vi "Pruebas con VISA.vi"() -> ()   [LabVIEW 2019]
uses:
  Controles/Amp_Frec.ctl
  <vilib>/Utility/error.llb/DialogType.ctl
  QMH_Support/Enqueue Message (Single).vi
  Varios/Globales.vi
  <vilib>/Utility/error.llb/Error Cluster From Error Code.vi
  <vilib>/ErrorRing/Error Ring.xnode
  QMH_Support/Message Queue.lvlib
  QMH_Support/User Event - Stop/User Event - Stop.lvlib
  DS360/DS360.lvlib
  K2002/K2002.lvlib
  CNT90/CNT90.lvlib
panel:
  in  "CNT90":refnum<visa-resource-name>
  in  "DS360":refnum<visa-resource-name>
  in  "K2002":refnum<visa-resource-name>
  in  "go_A":bool
  out "CNT90":i32
  out "K2002":i32
  out "DS360":i32
  out "Voltaje a generar":dbl(knob) scale=0.0..10.0
  out "error out":errorcluster
  in  "stop":bool
  in  "generar":bool
  in  "Voltaje a Generar":dbl(slide)=7.0649350649350655 scale=0.0..10.0
  out "voltMon":dbl format="%.2f"
  out "frecMon":dbl format="%.2f"
  # "Ensayo Eléctrico Ponderación A"
  # "Monitoreo"
  # "Frecuencia"
  # "Hz"
  # "Voltaje"
  # "mV"
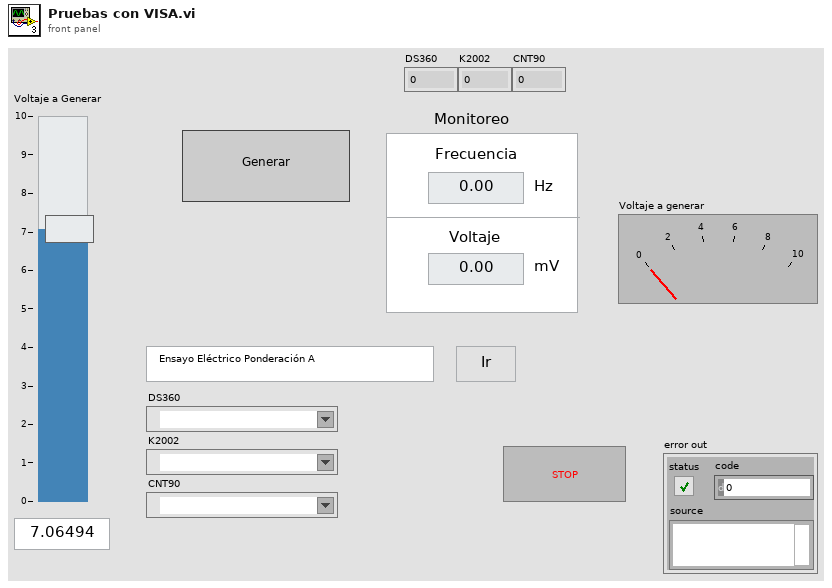
[diagram p1: front panel]
types:
  T1 = typedef "Message Queue.lvlib/All Message Queues.ctl" = cluster{"MHL":refnum<queue>, "DS360":refnum<queue>, "K2002":refnum<queue>, "CNT90":refnum<queue>}
  T2 = typedef "Amp_Frec.ctl" = cluster{"Ampl":dbl, "Frec":dbl}
  T3 = typedef "DialogType.ctl" = u16
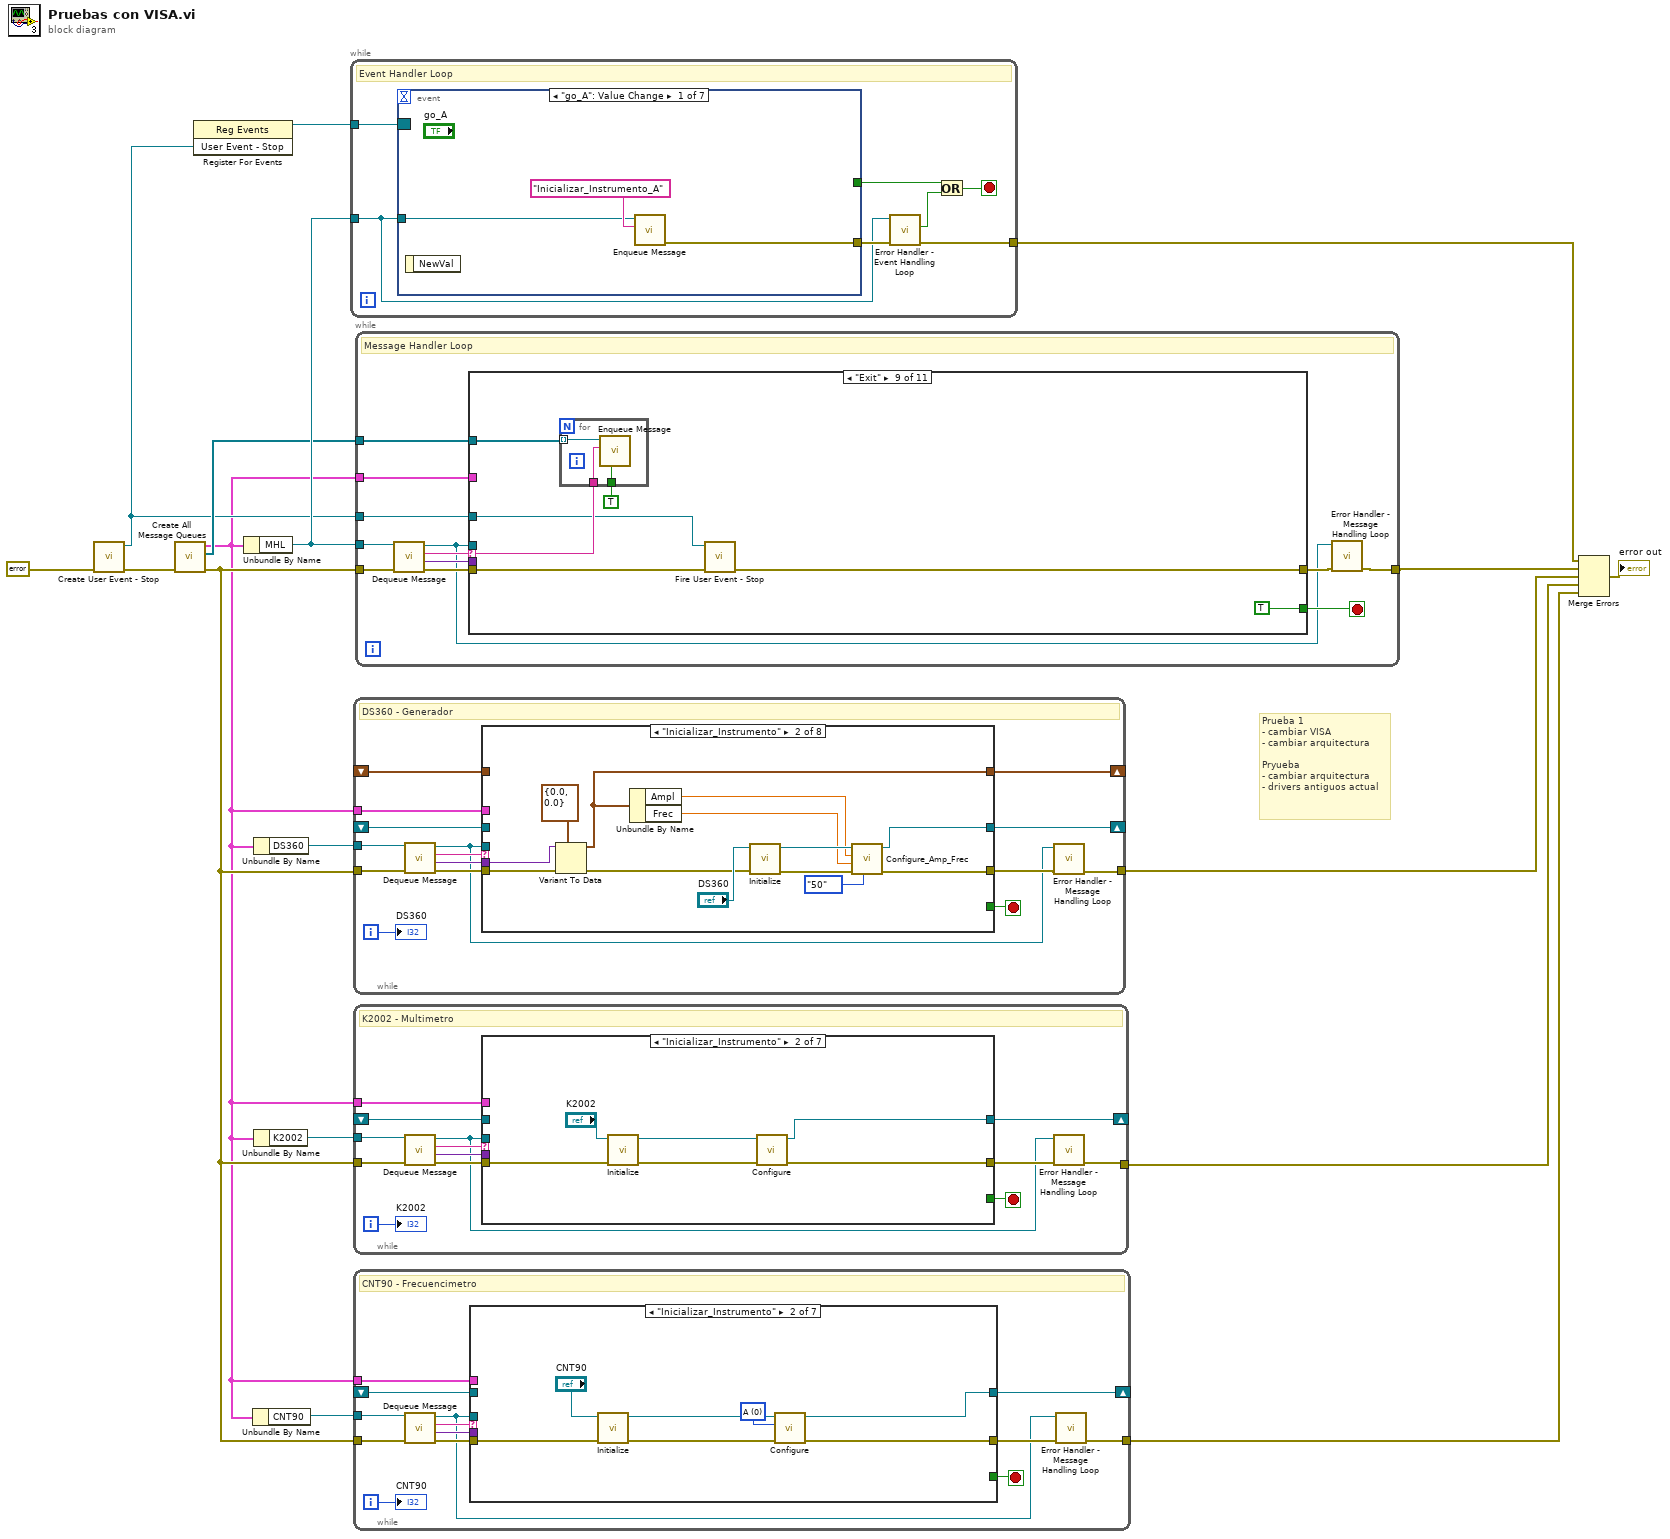
[diagram p0: block diagram]
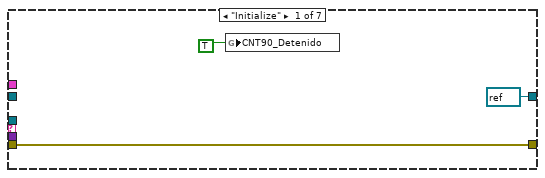
[diagram p2: hidden frame]
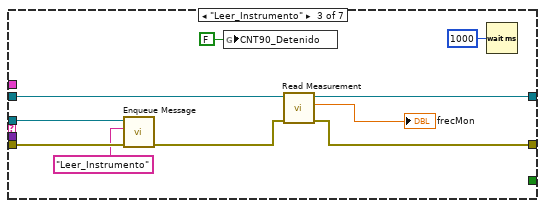
[diagram p3: hidden frame]
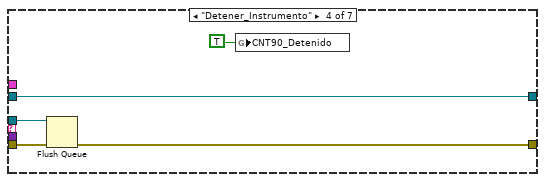
[diagram p4: hidden frame]
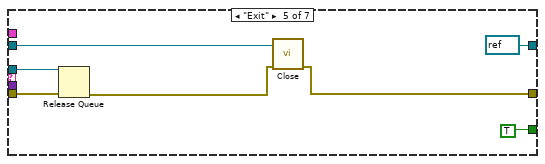
[diagram p5: hidden frame]
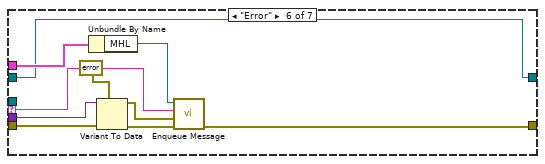
[diagram p6: hidden frame]
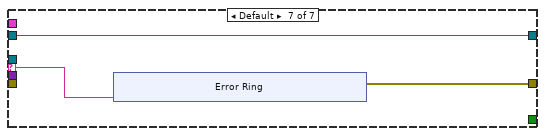
[diagram p7: hidden frame]
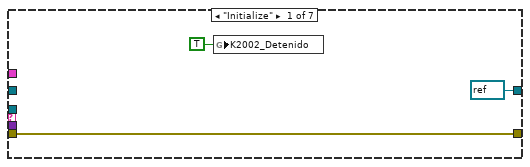
[diagram p8: hidden frame]
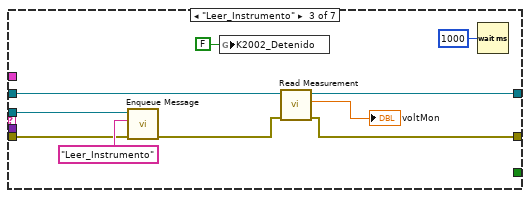
[diagram p9: hidden frame]
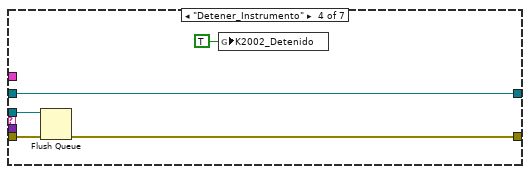
[diagram p10: hidden frame]
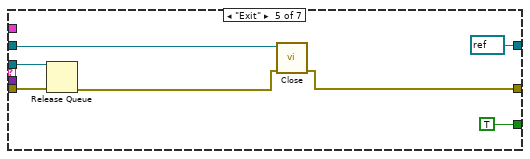
[diagram p11: hidden frame]
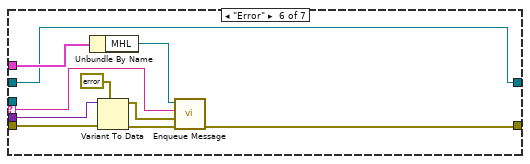
[diagram p12: hidden frame]
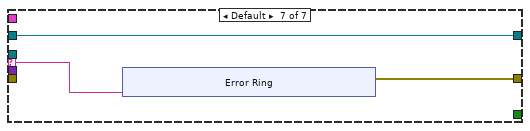
[diagram p13: hidden frame]
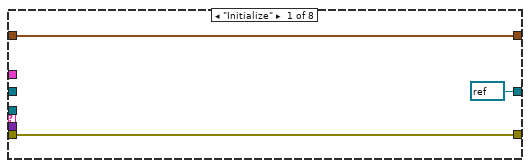
[diagram p14: hidden frame]
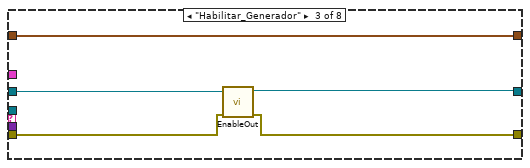
[diagram p15: hidden frame]
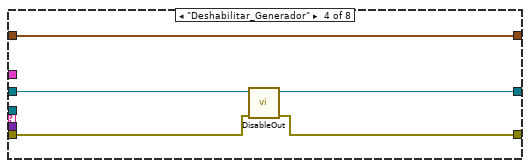
[diagram p16: hidden frame]
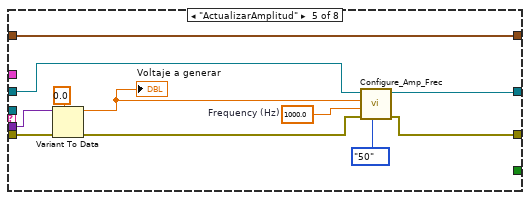
[diagram p17: hidden frame]
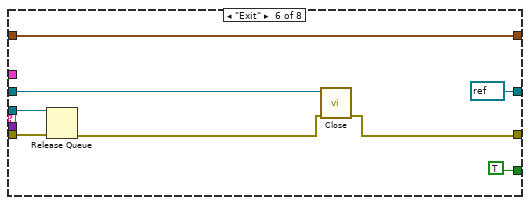
[diagram p18: hidden frame]
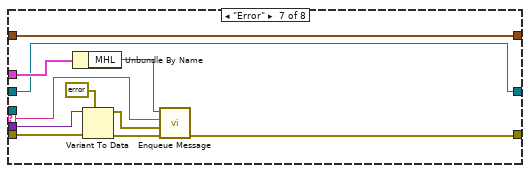
[diagram p19: hidden frame]
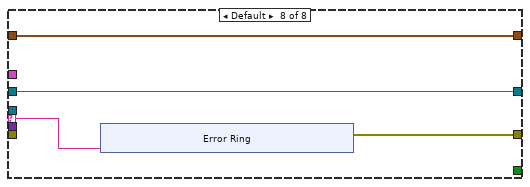
[diagram p20: hidden frame]
diagram:
  # "Prueba 1\n- cambiar VISA\n- cambiar arquitectura\n\nPryueba\n- cambiar arquitectura\n- drivers antiguos actual"
  n1 = call "Create User Event - Stop.vi"("error in (no error)"=errorcluster {"status"=FALSE, "code"=0, "source"=""}) -> ("error out"=w9:errorcluster, "User Event - Stop"=w8:refnum<user-event>)  [unwired: 9 in]
  n2 = call "Create All Message Queues.vi"("error in (no error)"=w9) -> ("error out"=w6:errorcluster, "Queues Array"=w11:refnum<queue>[], "Message Queues out"=w3:T1)  [unwired: 8 in]
  n3 = register-events(w8) -> (reference out=w7:refnum<event-registration>)  [unwired: 2 in, 1 out]
  n4 = Unbundle By Name(w3) -> ("MHL"=w17:refnum<queue>)
  n5 = Unbundle By Name(w3) -> ("CNT90"=w4:refnum<queue>)
  n6 = Unbundle By Name(w3) -> ("DS360"=w16:refnum<queue>)
  n7 = Unbundle By Name(w3) -> ("K2002"=w5:refnum<queue>)
  n8 = while {
    tunnel: w17 -> [w21]
    tunnel: [w22] -> w15
    tunnel: w7 -> [w24]
    stop <- w18 stop-if-true
    # "Event Handler Loop"
    n9 = event shown="[0] \"go_A\": Value Change" {
      selector: w24 -> [_ _ _ _ _ _ _]
      dyn-events: _ -> [_ _ _ _ _ _ _]
      timeout: _ -> [_ _ _ _ _ _ _]
      tunnel: w21 -> [w26 w29 w38 w46 w51 w59 _]
      tunnel: [w25 w28 w39 w45 w52 w57 _] -> w23
      tunnel: [_ _ _ _ _ _ TRUE] -> w20
      event "go_A": Value Change {
        n10 = event-data() -> ()  [unwired: 1 in, 1 out]
        n11 = call-poly "Enqueue Message.vi"("Message"="Inicializar_Instrumento_A" ("message"), "Message Queue"=w26) -> ("error out"=w25:errorcluster)  [unwired: 8 in, 1 out]
      }
      event "generar": Value Change {
        n12 = event-data() -> ("NewVal"=w30:bool)  [unwired: 1 in]
        n13 = Flush Queue(queue=w29) -> (queue out=w31:refnum<queue>, error out=w32:errorcluster)  [unwired: 1 in, 1 out]
        n14 = Select(t="iniciarGEN_A1" ("message"), s=w30, f="detenerGEN" ("message")) -> (s? t:f=w35:string)
        n15 = call-poly "Enqueue Message.vi"("Priority Message? (F)"=TRUE, "error in (no error)"=w32, "Message Data"="A1" ("message"), "Message"=w35, "Message Queue"=w31) -> ("error out"=w28:errorcluster)  [unwired: 5 in, 1 out]
      }
      event "Voltaje a Generar": Mouse Down {
        n16 = event-data() -> ()  [unwired: 1 in, 1 out]
        n17 = Flush Queue(queue=w38) -> (queue out=w40:refnum<queue>, error out=w41:errorcluster)  [unwired: 1 in, 1 out]
        n18 = call-poly "Enqueue Message.vi"("Priority Message? (F)"=TRUE, "error in (no error)"=w41, "Message"="Mouse_Down" ("message"), "Message Queue"=w40) -> ("error out"=w39:errorcluster)  [unwired: 6 in, 1 out]
      }
      event "Voltaje a Generar": Value Change {
        n19 = event-data() -> ("NewVal"=w44:dbl)  [unwired: 1 in]
        n20 = Flush Queue(queue=w46) -> (queue out=w47:refnum<queue>, error out=w48:errorcluster)  [unwired: 1 in, 1 out]
        n21 = call-poly "Enqueue Message.vi"("Priority Message? (F)"=TRUE, "error in (no error)"=w48, "Message Data"=w44, "Message"="EnviarVoltajeGEN" ("message"), "Message Queue"=w47) -> ("error out"=w45:errorcluster)  [unwired: 5 in, 1 out]
      }
      event "Voltaje a Generar": Mouse Up {
        n22 = event-data() -> ()  [unwired: 1 in, 1 out]
        n23 = Flush Queue(queue=w51) -> (queue out=w53:refnum<queue>, error out=w54:errorcluster)  [unwired: 1 in, 1 out]
        n24 = call-poly "Enqueue Message.vi"("Priority Message? (F)"=TRUE, "error in (no error)"=w54, "Message"="Reiniciar_Lectura" ("message"), "Message Queue"=w53) -> ("error out"=w52:errorcluster)  [unwired: 6 in, 1 out]
      }
      event "stop": Value Change {
        n25 = event-data() -> ()  [unwired: 1 in, 1 out]
        n26 = call-poly "Enqueue Message.vi"("Message"="Exit", "Message Queue"=w59) -> ("error out"=w57:errorcluster)  [unwired: 8 in, 1 out]
      }
      event User Event {
        n27 = event-data() -> ()  [unwired: 1 in, 1 out]
      }
    }
    n28 = call "Error Handler - Event Handling Loop.vi"("error in (no error)"=w23, "Message Queue"=w21) -> ("dup error in"=w22:errorcluster, "Error?"=w19:bool)  [unwired: 7 in, 1 out]
    n29 = Or(x=w20, y=w19) -> (x .or. y?=w18:bool)
  }
  n30 = while {
    tunnel: w16 -> [w75]
    tunnel: w6 -> [w74]
    tunnel: [w62] -> w13
    tunnel: w3 -> [w70]
    shift-right: [w67] -> _
    shift-left: _ -> [w66]
    shift-right: [w65] -> _
    shift-left: _ -> [w64]
    i -> [w68]
    stop <- w69 stop-if-true
    # "DS360 - Generador"
    n31 = call "Dequeue Message.vi"("error in (no error)"=w74, "Message Queue"=w75) -> ("error out"=w73:errorcluster, "Message Data"=w71:variant, "Message"=w72:string, "dup Message Queue"=w61:refnum<queue>)  [unwired: 6 in]
    n32 = case shown="\"Inicializar_Instrumento\"" w72 {
      selector: w72 -> [_ _ _ _ _ _ w124 w135]
      tunnel: w73 -> [w77 w91 w95 w98 w111 w120 w127 _]
      tunnel: w71 -> [_ w89 _ _ w110 _ w126 _]
      tunnel: w61 -> [_ _ _ _ _ w119 _ _]
      tunnel: [w77 w84 w94 w97 w107 w113 w123 w134] -> w63
      tunnel: w70 -> [_ _ _ _ _ _ w125 _]
      tunnel: [_ _ _ _ _ TRUE _ _] -> w69
      tunnel: [w78 w88 w96 w101 w109 w117 w122 w133] -> w67
      tunnel: w66 -> [w78 _ w96 w101 w109 w117 w122 w133]
      tunnel: [refnum<visa-resource-name> refnum ("VISA resource name out") w80 w92 w99 w106 refnum<visa-resource-name> refnum ("VISA resource name out") w121 w132] -> w65
      tunnel: w64 -> [_ _ w93 w100 w105 w116 w121 w132]
      frame "Initialize" {
      }
      frame "Inicializar_Instrumento" {
        n33 = Variant To Data(error in=w91, type=T2 {"Ampl"=0.0, "Frec"=0.0}, Variant=w89) -> (data=w88:T2, error out=w86:errorcluster)
        n34 = Unbundle By Name(w88) -> ("Ampl"=w82:dbl, "Frec"=w81:dbl)
        n35 = call "Initialize.vi"("error in (no error)"=w86, "VISA resource name"="DS360") -> ("error out"=w85:errorcluster, "VISA resource name out"=w83:refnum<visa-resource-name>)  [unwired: 8 in]
        n36 = call "Configure_Amp_Frec.vi"("Impedancia"=enum16{"50", "600", "HiZ"}."50", "error in (no error)"=w85, "Frequency (Hz)"=w81, "Amplitude (Vrms)"=w82, "VISA resource name"=w83) -> ("error out"=w84:errorcluster, "VISA resource name out"=w80:refnum<visa-resource-name>)  [unwired: 5 in]
      }
      frame "Habilitar_Generador" {
        n37 = call "EnableOut.vi"("error in (no error)"=w95, "VISA resource name"=w93) -> ("error out"=w94:errorcluster, "VISA resource name out"=w92:refnum<visa-resource-name>)  [unwired: 8 in]
      }
      frame "Deshabilitar_Generador" {
        n38 = call "DisableOut.vi"("error in (no error)"=w98, "VISA resource name"=w100) -> ("error out"=w97:errorcluster, "VISA resource name out"=w99:refnum<visa-resource-name>)  [unwired: 8 in]
      }
      frame "ActualizarAmplitud" {
        w103 = 1000.0  # Frequency (Hz)
        n39 = Variant To Data(error in=w111, type=0.0, Variant=w110) -> (data=w104:dbl, error out=w108:errorcluster)
        "Voltaje a generar" <- w104
        n40 = call "Configure_Amp_Frec.vi"("Impedancia"=enum16{"50", "600", "HiZ"}."50", "error in (no error)"=w108, "Frequency (Hz)"=w103, "Amplitude (Vrms)"=w104, "VISA resource name"=w105) -> ("error out"=w107:errorcluster, "VISA resource name out"=w106:refnum<visa-resource-name>)  [unwired: 5 in]
      }
      frame "Exit" {
        n41 = Release Queue(queue=w119, error in (no error)=w120) -> (error out=w114:errorcluster)  [unwired: 1 in, 2 out]
        n42 = call "Close.vi"("error in (no error)"=w114, "VISA resource name"=w116) -> ("error out"=w113:errorcluster)  [unwired: 9 in]
      }
      frame "Error" {
        n43 = Unbundle By Name(w125) -> ("MHL"=w128:refnum<queue>)
        n44 = Variant To Data(error in=w127, type=errorcluster {"status"=FALSE, "code"=0, "source"=""} ("error constant"), Variant=w126) -> (data=w129:errorcluster, error out=w130:errorcluster)
        n45 = call-poly "Enqueue Message.vi"("error in (no error)"=w130, "Message Data"=w129, "Message"=w124, "Message Queue"=w128) -> ("error out"=w123:errorcluster)  [unwired: 6 in, 1 out]
      }
      frame Default {
        n46 = xnode "Error Ring"("parameter 0"=w135) -> ("error out"=w134:errorcluster)
      }
    }
    n47 = call "Error Handler - Message Handling Loop.vi"("error in (no error)"=w63, "Message Queue"=w61) -> ("dup error in"=w62:errorcluster)  [unwired: 8 in, 1 out]
    "DS360" <- w68
  }
  n48 = while {
    tunnel: w5 -> [w155]
    tunnel: w6 -> [w154]
    tunnel: w3 -> [w150]
    shift-right: [w147] -> _
    shift-left: _ -> [w146]
    tunnel: [w144] -> w2
    i -> [w148]
    stop <- w149 stop-if-true
    # "K2002 - Multimetro"
    n49 = call "Dequeue Message.vi"("error in (no error)"=w154, "Message Queue"=w155) -> ("error out"=w153:errorcluster, "Message Data"=w151:variant, "Message"=w152:string, "dup Message Queue"=w143:refnum<queue>)  [unwired: 6 in]
    n50 = case shown="\"Inicializar_Instrumento\"" w152 {
      selector: w152 -> [_ _ _ _ _ w189 w199]
      tunnel: w153 -> [w157 w164 w172 w179 w186 w192 _]
      tunnel: w151 -> [_ _ _ _ _ w191 _]
      tunnel: w143 -> [_ _ w171 w177 w185 _ _]
      tunnel: [w157 w162 w168 w178 w181 w188 w198] -> w145
      tunnel: w150 -> [_ _ _ _ _ w190 _]
      tunnel: [_ _ _ _ TRUE _ _] -> w149
      tunnel: [refnum<visa-resource-name> refnum ("VISA resource name out") w160 w166 w175 refnum<visa-resource-name> refnum ("VISA resource name out") w187 w197] -> w147
      tunnel: w146 -> [_ _ w167 w175 w182 w187 w197]
      frame "Initialize" {
        n51 = global write "Globales.vi" "K2002_Detenido"(TRUE ("K2002_Detenido")) -> ()
      }
      frame "Inicializar_Instrumento" {
        n52 = call "Initialize.vi"("error in (no error)"=w164, "VISA resource name"="K2002") -> ("error out"=w163:errorcluster, "VISA resource name out"=w161:refnum<visa-resource-name>)  [unwired: 8 in]
        n53 = call "Configure.vi"("error in (no error)"=w163, "VISA resource name"=w161) -> ("error out"=w162:errorcluster, "VISA resource name out"=w160:refnum<visa-resource-name>)  [unwired: 8 in]
      }
      frame "Leer_Instrumento" {
        n54 = call-poly "Enqueue Message.vi"("error in (no error)"=w172, "Message"="Leer_Instrumento", "Message Queue"=w171) -> ("error out"=w169:errorcluster)  [unwired: 7 in, 1 out]
        n55 = global write "Globales.vi" "K2002_Detenido"(FALSE ("K2002_Detenido")) -> ()
        n56 = call "Read Measurement.vi"("error in (no error)"=w169, "VISA resource name"=w167) -> ("error out"=w168:errorcluster, "Measurement"=→"voltMon":dbl, "VISA resource name out"=w166:refnum<visa-resource-name>)  [unwired: 7 in]
        n57 = Wait (ms)(milliseconds to wait=u32 1000) -> ()  [unwired: 1 out]
      }
      frame "Detener_Instrumento" {
        n58 = Flush Queue(queue=w177, error in (no error)=w179) -> (error out=w178:errorcluster)  [unwired: 2 out]
        n59 = global write "Globales.vi" "K2002_Detenido"(TRUE ("K2002_Detenido")) -> ()
      }
      frame "Exit" {
        n60 = Release Queue(queue=w185, error in (no error)=w186) -> (error out=w183:errorcluster)  [unwired: 1 in, 2 out]
        n61 = call "Close.vi"("error in (no error)"=w183, "VISA resource name"=w182) -> ("error out"=w181:errorcluster)  [unwired: 9 in]
      }
      frame "Error" {
        n62 = Unbundle By Name(w190) -> ("MHL"=w193:refnum<queue>)
        n63 = Variant To Data(error in=w192, type=errorcluster {"status"=FALSE, "code"=0, "source"=""} ("error constant"), Variant=w191) -> (data=w194:errorcluster, error out=w195:errorcluster)
        n64 = call-poly "Enqueue Message.vi"("error in (no error)"=w195, "Message Data"=w194, "Message"=w189, "Message Queue"=w193) -> ("error out"=w188:errorcluster)  [unwired: 6 in, 1 out]
      }
      frame Default {
        n65 = xnode "Error Ring"("parameter 0"=w199) -> ("error out"=w198:errorcluster)
      }
    }
    n66 = call "Error Handler - Message Handling Loop.vi"("error in (no error)"=w145, "Message Queue"=w143) -> ("dup error in"=w144:errorcluster)  [unwired: 8 in, 1 out]
    "K2002" <- w148
  }
  n67 = while {
    tunnel: w4 -> [w219]
    tunnel: w6 -> [w218]
    tunnel: w3 -> [w214]
    shift-right: [w211] -> _
    shift-left: _ -> [w210]
    tunnel: [w208] -> w1
    i -> [w212]
    stop <- w213 stop-if-true
    # "CNT90 - Frecuencimetro"
    n68 = call "Dequeue Message.vi"("error in (no error)"=w218, "Message Queue"=w219) -> ("error out"=w217:errorcluster, "Message Data"=w215:variant, "Message"=w216:string, "dup Message Queue"=w207:refnum<queue>)  [unwired: 6 in]
    n69 = case shown="\"Inicializar_Instrumento\"" w216 {
      selector: w216 -> [_ _ _ _ _ w254 w264]
      tunnel: w217 -> [w222 w229 w239 w244 w251 w257 _]
      tunnel: w215 -> [_ _ _ _ _ w256 _]
      tunnel: w207 -> [_ _ w235 w242 w250 _ _]
      tunnel: [w222 w227 w238 w243 w245 w253 w263] -> w209
      tunnel: w214 -> [_ _ _ _ _ w255 _]
      tunnel: [_ _ _ _ TRUE _ _] -> w213
      tunnel: [refnum<visa-resource-name> refnum ("VISA resource name out") w223 w230 w240 refnum<visa-resource-name> refnum ("VISA resource name out") w252 w262] -> w211
      tunnel: w210 -> [_ _ w231 w240 w247 w252 w262]
      frame "Initialize" {
        n70 = global write "Globales.vi" "CNT90_Detenido"(TRUE ("CNT90_Detenido")) -> ()
      }
      frame "Inicializar_Instrumento" {
        w224 = 0 items=["A", "B"] ("Channel  1")
        n71 = call "Initialize.vi"("error in (no error)"=w229, "VISA resource name"="CNT90") -> ("error out"=w228:errorcluster, "VISA resource name out"=w225:refnum<visa-resource-name>)  [unwired: 8 in]
        n72 = call "Configure.vi"("error in (no error)"=w228, "Channel  1"=w224, "VISA resource name"=w225) -> ("error out"=w227:errorcluster, "VISA resource name out"=w223:refnum<visa-resource-name>)  [unwired: 7 in]
      }
      frame "Leer_Instrumento" {
        n73 = call-poly "Enqueue Message.vi"("error in (no error)"=w239, "Message"="Leer_Instrumento", "Message Queue"=w235) -> ("error out"=w236:errorcluster)  [unwired: 7 in, 1 out]
        n74 = global write "Globales.vi" "CNT90_Detenido"(FALSE ("CNT90_Detenido")) -> ()
        n75 = call "Read Measurement.vi"("error in (no error)"=w236, "VISA resource name"=w231) -> ("error out"=w238:errorcluster, "Measurement"=→"frecMon":dbl, "VISA resource name out"=w230:refnum<visa-resource-name>)  [unwired: 7 in]
        n76 = Wait (ms)(milliseconds to wait=u32 1000) -> ()  [unwired: 1 out]
      }
      frame "Detener_Instrumento" {
        n77 = Flush Queue(queue=w242, error in (no error)=w244) -> (error out=w243:errorcluster)  [unwired: 2 out]
        n78 = global write "Globales.vi" "CNT90_Detenido"(TRUE ("CNT90_Detenido")) -> ()
      }
      frame "Exit" {
        n79 = Release Queue(queue=w250, error in (no error)=w251) -> (error out=w246:errorcluster)  [unwired: 1 in, 2 out]
        n80 = call "Close.vi"("error in (no error)"=w246, "VISA resource name"=w247) -> ("error out"=w245:errorcluster)  [unwired: 9 in]
      }
      frame "Error" {
        n81 = Unbundle By Name(w255) -> ("MHL"=w258:refnum<queue>)
        n82 = Variant To Data(error in=w257, type=errorcluster {"status"=FALSE, "code"=0, "source"=""} ("error constant"), Variant=w256) -> (data=w259:errorcluster, error out=w260:errorcluster)
        n83 = call-poly "Enqueue Message.vi"("error in (no error)"=w260, "Message Data"=w259, "Message"=w254, "Message Queue"=w258) -> ("error out"=w253:errorcluster)  [unwired: 6 in, 1 out]
      }
      frame Default {
        n84 = xnode "Error Ring"("parameter 0"=w264) -> ("error out"=w263:errorcluster)
      }
    }
    n85 = call "Error Handler - Message Handling Loop.vi"("error in (no error)"=w209, "Message Queue"=w207) -> ("dup error in"=w208:errorcluster)  [unwired: 8 in, 1 out]
    "CNT90" <- w212
  }
  n86 = while {
    tunnel: w17 -> [w283]
    tunnel: w6 -> [w282]
    tunnel: [w274] -> w14
    tunnel: w11 -> [w278]
    tunnel: w8 -> [w276]
    tunnel: w3 -> [w272]
    stop <- w277 stop-if-true
    # "Message Handler Loop"
    n87 = call "Dequeue Message.vi"("error in (no error)"=w282, "Message Queue"=w283) -> ("error out"=w279:errorcluster, "Message Data"=w280:variant, "Message"=w281:string, "dup Message Queue"=w273:refnum<queue>)  [unwired: 6 in]
    n88 = case shown="\"Exit\"" w281 {
      selector: w281 -> [_ _ _ _ _ _ _ _ w366 _ w381]
      tunnel: w280 -> [_ _ _ _ w325 _ w349 _ _ w371 _]
      tunnel: w279 -> [w285 w297 w308 w313 w326 w340 w350 w358 w363 w374 _]
      tunnel: w273 -> [_ _ _ _ _ _ _ _ _ w372 _]
      tunnel: [w284 w295 w299 w309 w320 w334 w344 w356 w362 w373 w380] -> w275
      tunnel: w278 -> [_ _ _ _ _ _ _ _ w367 _ _]
      tunnel: [_ _ _ _ _ _ _ _ TRUE _ _] -> w277
      tunnel: w276 -> [_ _ _ _ _ _ _ _ w361 _ _]
      tunnel: w272 -> [_ w293 w307 w312 w324 w339 w348 w357 _ _ _]
      frame "Initialize" {
        n89 = invoke class="VI" method="Default Vals.Reinit All"(error in=w285) -> (error out=w284:errorcluster)  [unwired: 2 in, 2 out]
      }
      frame "Inicializar_Instrumento_A" {
        w294 = "Inicializar_Instrumento" ("Message")
        n90 = Unbundle By Name(w293) -> ("CNT90"=w290:refnum<queue>, "K2002"=w291:refnum<queue>, "DS360"=w292:refnum<queue>)
        n91 = local read "Voltaje a Generar"() -> (w287:dbl)
        n92 = Bundle By Name(cluster=T2 {"Ampl"=0.0, "Frec"=0.0}, "Ampl"=w287, "Frec"=1000.0) -> (w288:T2)
        n93 = call-poly "Enqueue Message.vi"("error in (no error)"=w297, "Message Data"=w288, "Message"=w294, "Message Queue"=w292) -> ("error out"=w298:errorcluster)  [unwired: 6 in, 1 out]
        n94 = call-poly "Enqueue Message.vi"("error in (no error)"=w298, "Message"=w294, "Message Queue"=w291) -> ("error out"=w296:errorcluster)  [unwired: 7 in, 1 out]
        n95 = call-poly "Enqueue Message.vi"("error in (no error)"=w296, "Message"=w294, "Message Queue"=w290) -> ("error out"=w295:errorcluster)  [unwired: 7 in, 1 out]
      }
      frame "iniciarGEN_A1" {
        w302 = "Leer_Instrumento" ("Message")
        n96 = Unbundle By Name(w307) -> ("CNT90"=w303:refnum<queue>, "K2002"=w304:refnum<queue>, "DS360"=w306:refnum<queue>)
        n97 = call-poly "Enqueue Message.vi"("error in (no error)"=w308, "Message"="Habilitar_Generador", "Message Queue"=w306) -> ("error out"=w301:errorcluster)  [unwired: 7 in, 1 out]
        n98 = call-poly "Enqueue Message.vi"("error in (no error)"=w301, "Message"=w302, "Message Queue"=w304) -> ("error out"=w300:errorcluster)  [unwired: 7 in, 1 out]
        n99 = call-poly "Enqueue Message.vi"("error in (no error)"=w300, "Message"=w302, "Message Queue"=w303) -> ("error out"=w299:errorcluster)  [unwired: 7 in, 1 out]
      }
      frame "Mouse_Down" {
        w314 = TRUE ("Priority Message? (F)")
        w315 = "Detener_Instrumento" ("Message")
        n100 = Unbundle By Name(w312) -> ("CNT90"=w310:refnum<queue>, "K2002"=w311:refnum<queue>)
        n101 = call-poly "Enqueue Message.vi"("Priority Message? (F)"=w314, "error in (no error)"=w313, "Message"=w315, "Message Queue"=w311) -> ("error out"=w316:errorcluster)  [unwired: 6 in, 1 out]
        n102 = call-poly "Enqueue Message.vi"("Priority Message? (F)"=w314, "error in (no error)"=w316, "Message"=w315, "Message Queue"=w310) -> ("error out"=w309:errorcluster)  [unwired: 6 in, 1 out]
      }
      frame "EnviarVoltajeGEN" {
        n103 = Variant To Data(error in=w326, type=0.0, Variant=w325) -> (data=w321:dbl, error out=w322:errorcluster)
        n104 = Unbundle By Name(w324) -> ("DS360"=w323:refnum<queue>)
        n105 = global read "Globales.vi" "CNT90_Detenido"() -> (w318:bool)
        n106 = global read "Globales.vi" "K2002_Detenido"() -> (w319:bool)
        n107 = And(x=w319, y=w318) -> (x .and. y?=w317:bool)
        n108 = case shown="True" w317 {
          tunnel: w323 -> [_ w332]
          tunnel: w322 -> [w328 w331]
          tunnel: w321 -> [_ w330]
          tunnel: [w328 w329] -> w320
          frame False {
          }
          frame True {
            n109 = call-poly "Enqueue Message.vi"("error in (no error)"=w331, "Message Data"=w330, "Message"="ActualizarAmplitud", "Message Queue"=w332) -> ("error out"=w329:errorcluster)  [unwired: 6 in, 1 out]
          }
        }
      }
      frame "Reiniciar_Lectura" {
        w336 = "Leer_Instrumento" ("Message")
        n110 = Unbundle By Name(w339) -> ("CNT90"=w337:refnum<queue>, "K2002"=w338:refnum<queue>)
        n111 = call-poly "Enqueue Message.vi"("error in (no error)"=w340, "Message"=w336, "Message Queue"=w338) -> ("error out"=w335:errorcluster)  [unwired: 7 in, 1 out]
        n112 = call-poly "Enqueue Message.vi"("error in (no error)"=w335, "Message"=w336, "Message Queue"=w337) -> ("error out"=w334:errorcluster)  [unwired: 7 in, 1 out]
      }
      frame "Leer_Instrumento" {
        w343 = TRUE ("Priority Message? (F)")
        w345 = "Leer_Instrumento" ("Message")
        n113 = Variant To Data(error in=w350, type=0.0, Variant=w349) -> (error out=w347:errorcluster)  [unwired: 1 out]
        n114 = Unbundle By Name(w348) -> ("K2002"=w342:refnum<queue>, "CNT90"=w341:refnum<queue>)  [unwired: 1 out]
        n115 = call-poly "Enqueue Message.vi"("Priority Message? (F)"=w343, "error in (no error)"=w347, "Message"=w345, "Message Queue"=w341) -> ("error out"=w346:errorcluster)  [unwired: 6 in, 1 out]
        n116 = call-poly "Enqueue Message.vi"("Priority Message? (F)"=w343, "error in (no error)"=w346, "Message"=w345, "Message Queue"=w342) -> ("error out"=w344:errorcluster)  [unwired: 6 in, 1 out]
      }
      frame "detenerGEN" {
        w352 = "Detener_Instruemento" ("Message")
        w355 = 0.0 ("frecMon")
        n117 = Unbundle By Name(w357) -> ("CNT90"=w353:refnum<queue>, "K2002"=w354:refnum<queue>, "DS360"=w360:refnum<queue>)
        n118 = call-poly "Enqueue Message.vi"("error in (no error)"=w358, "Message"="Deshabilitar_Generador", "Message Queue"=w360) -> ("error out"=w356:errorcluster)  [unwired: 7 in, 1 out]
        n119 = call-poly "Enqueue Message.vi"("Message"=w352, "Message Queue"=w354) -> ()  [unwired: 8 in, 2 out]
        n120 = call-poly "Enqueue Message.vi"("Message"=w352, "Message Queue"=w353) -> ()  [unwired: 8 in, 2 out]
        n121 = local write "frecMon"(w355) -> ()
        n122 = local write "voltMon"(w355) -> ()
      }
      frame "Exit" {
        n123 = for {
          tunnel: w367 -> [w370] mode=indexing
          tunnel: w366 -> [w369]
          tunnel: TRUE -> [w368]
          n124 = call-poly "Enqueue Message.vi"("Priority Message? (F)"=w368, "Message"=w369, "Message Queue"=w370) -> ()  [unwired: 7 in, 2 out]
        }
        n125 = call "Fire User Event - Stop.vi"("error in (no error)"=w363, "User Event - Stop"=w361) -> ("error out"=w362:errorcluster)  [unwired: 9 in]
      }
      frame "Error" {
        w378 = T3 1 items=["no dialog", "OK message", "continue or stop message", "OK message + warnings", "continue/stop + warnings"] ("type of dialog (OK msg:1)")
        n126 = Variant To Data(error in=w374, type=errorcluster {"status"=FALSE, "code"=0, "source"=""} ("error out"), Variant=w371) -> (data=w376:errorcluster, error out=w375:errorcluster)
        n127 = call <vilib>:"Simple Error Handler.vi"("type of dialog (OK msg:1)"=w378, "error in (no error)"=w376) -> ()  [unwired: 3 in, 5 out]
        n128 = call-poly "Enqueue Message.vi"("error in (no error)"=w375, "Message"="Exit", "Message Queue"=w372) -> ("error out"=w373:errorcluster)  [unwired: 7 in, 1 out]
      }
      frame Default {
        n129 = xnode "Error Ring"("parameter 0"=w381) -> ("error out"=w380:errorcluster)
      }
    }
    n130 = call "Error Handler - Message Handling Loop.vi"("error in (no error)"=w275, "Message Queue"=w273) -> ("dup error in"=w274:errorcluster)  [unwired: 8 in, 1 out]
  }
  n131 = Merge Errors(w15, w14, w13, w2, w1) -> (→"error out":errorcluster)
